vi "Write Setpoints.vi"(8 "error in":errorcluster, 10 "Setpoints":sgl[](array[numeric]), 11 "AlicatCommBank in":refnum<class "AlicatCommBank.lvclass">) -> (0 "error out":errorcluster, 3 "AlicatCommBank out":refnum<class "AlicatCommBank.lvclass">)   [LabVIEW 2015, in "Alicat.lvlib" / "AlicatCommBank.lvclass"]
doc: "Write the setpoints to an Alicat controller. If any of the devices are not controllers, no attempt is made to write a setpoint value to that device. There should be the same number of setpoints as there are controllers, no more no less."
uses:
  AlicatCommBank.lvclass
  Alicat Controller/Alicat Controller.lvclass
  AlicatCommBank.lvclass/AlicatCommBank.ctl
  Alicat.lvclass
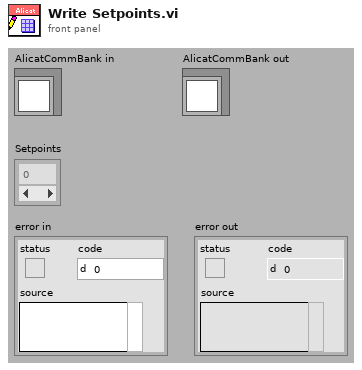
[diagram p1: front panel]
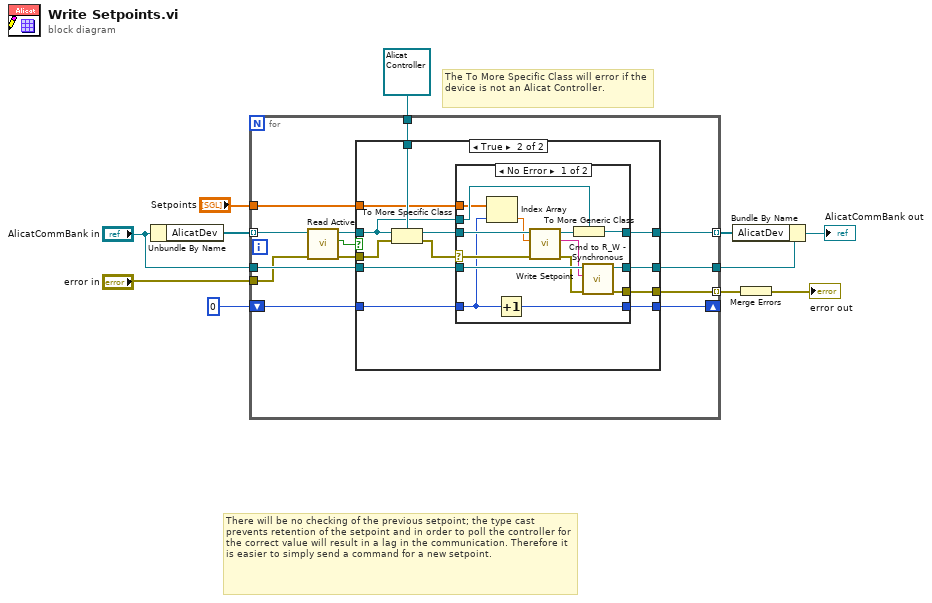
[diagram p0: block diagram]
diagram:
  # "There will be no checking of the previous setpoint; the type cast prevents retention of the setpoint and in order to poll the controller for the correct value will result in a lag in the communication. Therefore it is easier to simply send a command for a new setpoint."
  # "The To More Specific Class will error if the device is not an Alicat Controller."
  n1 = Unbundle By Name("AlicatCommBank in") -> ("AlicatDev"=w10:refnum<class "Alicat.lvclass">[])
  n2 = for {
    tunnel: "Setpoints" -> [w17]
    tunnel: "AlicatCommBank in" -> [w24]
    tunnel: [w23] -> w5
    tunnel: [w22] -> w3 mode=indexing
    tunnel: "error in" -> [w14]
    tunnel: w10 -> [w16] mode=indexing
    tunnel: refnum<class "Alicat Controller.lvclass"> refnum ("Alicat Controller.lvclass") -> [w21]
    shift-right: [w19] -> _
    shift-left: 0 -> [w20]
    tunnel: [w18] -> w4 mode=indexing
    n3 = call "Read Active.vi"("error in"=w14, "Alicat in"=w16) -> ("error out"=w13:errorcluster, "Active?"=w12:bool, "Alicat out"=w15:refnum<class "Alicat.lvclass">)  [unwired: 7 in]
    n4 = case shown="True" w12 {
      tunnel: w24 -> [w27 w40]
      tunnel: [w27 w39] -> w23
      tunnel: [w26 w38] -> w22
      tunnel: w21 -> [_ w37]
      tunnel: w20 -> [w25 w34]
      tunnel: [w25 w33] -> w19
      tunnel: [w28 w32] -> w18
      tunnel: w17 -> [_ w31]
      tunnel: w15 -> [w28 w30]
      tunnel: w13 -> [w26 w29]
      frame False {
      }
      frame True {
        n5 = To More Specific Class(target class=w37, reference=w30, error in=w29) -> (specific class reference=w36:refnum<class "Alicat Controller.lvclass">, error out=w35:errorcluster)
        n6 = case shown="No Error" w35 {
          selector: w35 -> [w49 _]
          tunnel: w31 -> [w46 _]
          tunnel: w40 -> [w54 w56]
          tunnel: [w53 w56] -> w39
          tunnel: [w52 _] -> w38
          tunnel: w36 -> [w50 _]
          tunnel: w34 -> [w44 w57]
          tunnel: [w51 w57] -> w33
          tunnel: [w48 w55] -> w32
          tunnel: w30 -> [w47 w55]
          frame No Error {
            n7 = Index Array(array=w46, index=w44) -> (element=w45:sgl)
            n8 = Increment(x=w44) -> (x+1=w51:i32)
            n9 = call "Write Setpoint.vi"("error in"=w49, "Setpoint"=w45, "Alicat Controller in"=w50) -> ("error out"=w42:errorcluster, "SPStr"=w43:string, "Alicat Controller out"=w41:refnum<class "Alicat Controller.lvclass">)  [unwired: 6 in]
            n10 = To More Generic Class(target class=w47, reference=w41) -> (generic class reference=w48:refnum<class "Alicat.lvclass">)
            n11 = call-dynamic "Cmd to R_W - Synchronous.vi"("error in"=w42, "write buffer"=w43, "Serial IO in"=w54) -> ("error out"=w52:errorcluster, "Serial IO out"=w53:refnum<class "AlicatCommBank.lvclass">)  [unwired: 6 in, 1 out]
          }
          frame Error {
            # "Not a controller"
          }
        }
      }
    }
  }
  n12 = Bundle By Name(cluster=w5, "AlicatDev"=w4) -> (→"AlicatCommBank out":refnum<class "AlicatCommBank.lvclass">)
  n13 = Merge Errors(w3) -> (→"error out":errorcluster)
